vi "数据处理整合 (子VI).vi"(11 "枚举":enum16{"实时数据排序", "小时数据排序"}(ring)) -> (3 "已排序的数组":string[](array[string]))   [LabVIEW 2016, in "数据传输系统.lvlib"]
uses:
  <userlib>/_OpenG.lib/array/array.llb/Remove Duplicates from 1D Array (String)__ogtk.vi
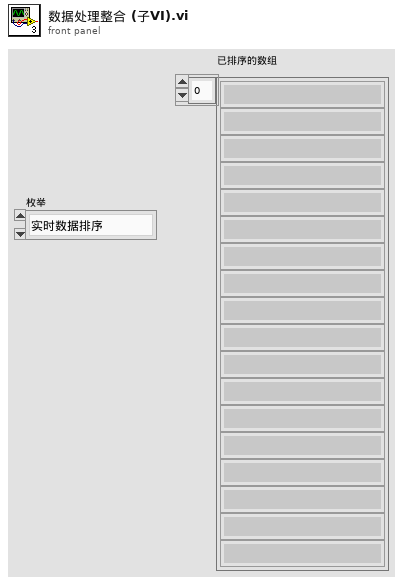
[diagram p1: front panel]
types:
  T1 = cluster{"PH":string[][], "CODCr":string[][], "氨氮":string[][], "CODMn":string[][], "总氮":string[][], "总磷":string[][], "电导率":string[][], "水温":string[][], "DO":string[][], "浊度":string[][], "叶绿素":string[][], "藻密度":string[][], "铜":string[][], "盐度":string[][], "水位":string[][], "流速":string[][], "瞬时流量":string[][], "累积流量":string[][], "亚硝酸盐":string[][], "硫化物":string[][], "ORP":string[][], "铅":string[][], "镉":string[][], "锌":string[][], "镍":string[][], "锰":string[][], "汞":string[][]}
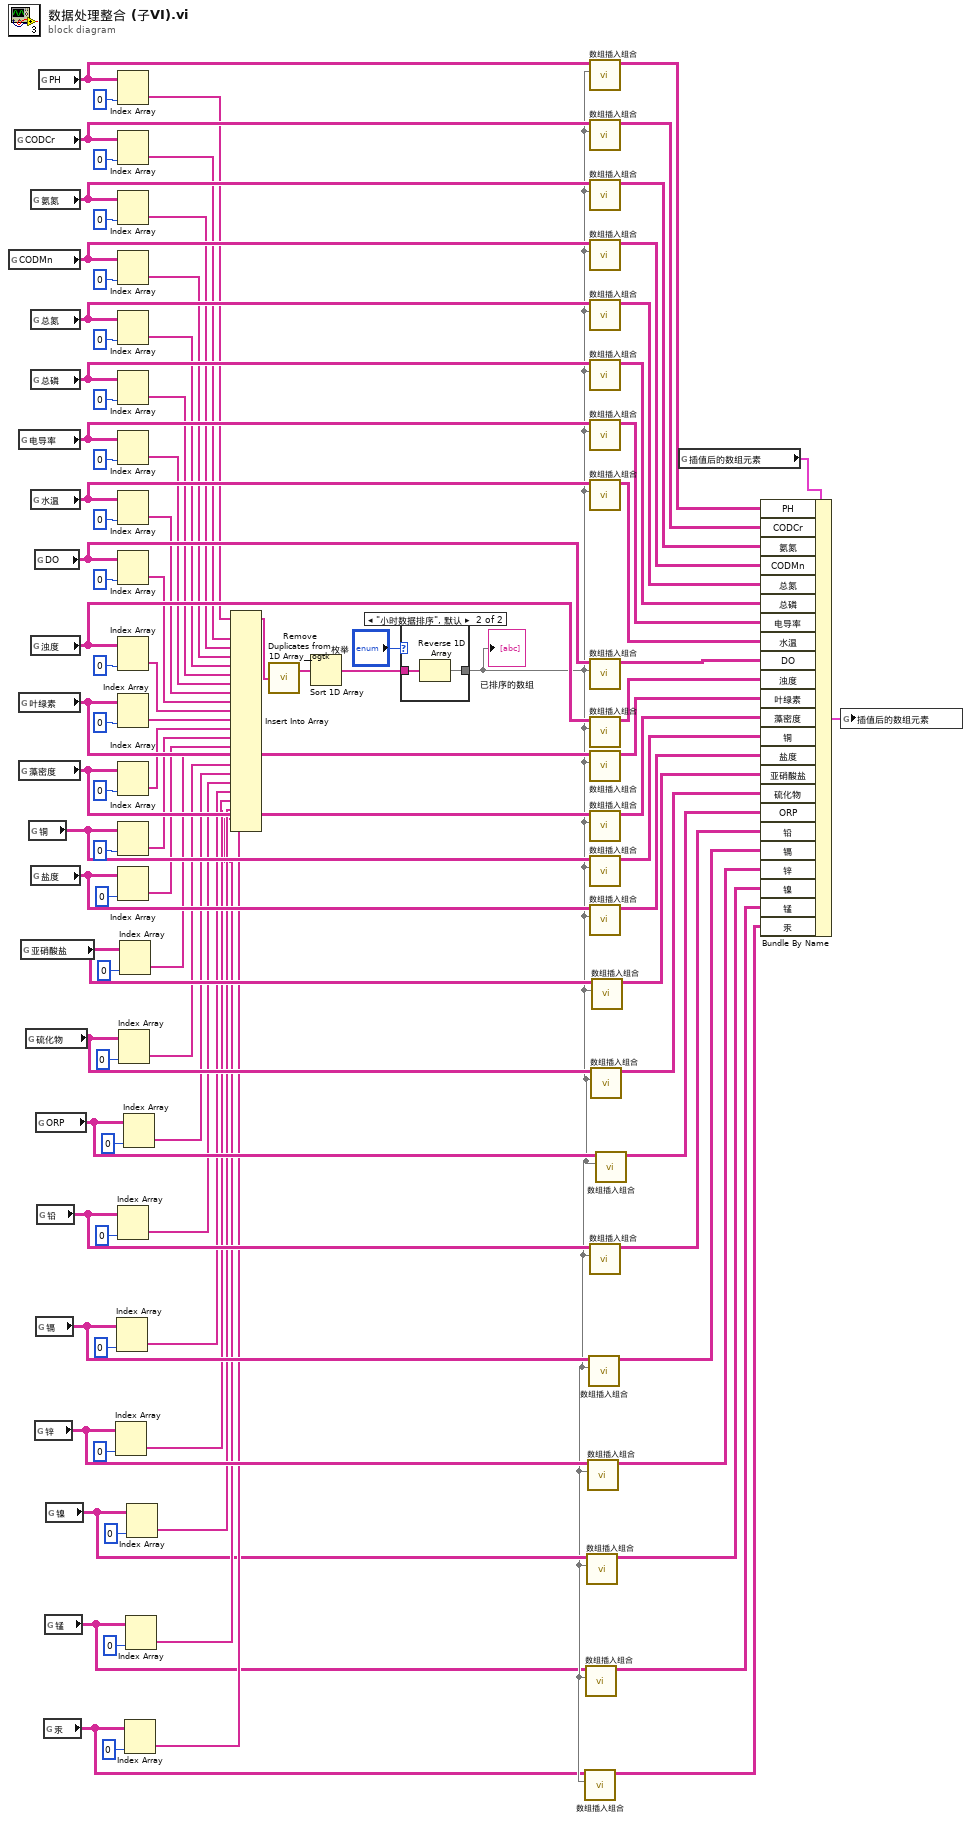
[diagram p0: block diagram]
diagram:
  n1 = global read "全局 所有参数.vi" "CODMn"() -> (w80:string[][])
  n2 = global read "全局 所有参数.vi" "CODCr"() -> (w78:string[][])
  n3 = global read "全局 所有参数.vi" "电导率"() -> (w83:string[][])
  n4 = global read "全局 所有参数.vi" "叶绿素"() -> (w87:string[][])
  n5 = global read "全局 所有参数.vi" "藻密度"() -> (w88:string[][])
  n6 = global read "全局 所有参数.vi" "亚硝酸盐"() -> (w37:string[][])
  n7 = global read "全局 所有参数.vi" "硫化物"() -> (w36:string[][])
  n8 = global read "全局 所有参数.vi" "铜"() -> (w47:string[][])
  n9 = global read "全局 所有参数.vi" "氨氮"() -> (w79:string[][])
  n10 = global read "全局 所有参数.vi" "总氮"() -> (w81:string[][])
  n11 = global read "全局 所有参数.vi" "总磷"() -> (w82:string[][])
  n12 = global read "全局 所有参数.vi" "水温"() -> (w84:string[][])
  n13 = global read "全局 所有参数.vi" "浊度"() -> (w86:string[][])
  n14 = global read "全局 所有参数.vi" "盐度"() -> (w46:string[][])
  n15 = global read "全局 所有参数.vi" "DO"() -> (w85:string[][])
  n16 = global read "全局 所有参数.vi" "锌"() -> (w21:string[][])
  n17 = global read "全局 所有参数.vi" "ORP"() -> (w33:string[][])
  n18 = global read "全局 所有参数.vi" "镉"() -> (w22:string[][])
  n19 = global read "全局 所有参数.vi" "铅"() -> (w25:string[][])
  n20 = global read "全局 所有参数.vi" "PH"() -> (w76:string[][])
  n21 = global read "全局 所有参数.vi" "汞"() -> (w4:string[][])
  n22 = global read "全局 所有参数.vi" "锰"() -> (w5:string[][])
  n23 = global read "全局 所有参数.vi" "镍"() -> (w7:string[][])
  n24 = Index Array(array=w21, index (col)=0 ("索引 (行)")) -> (element=w14:string[])  [unwired: 1 in]
  n25 = Index Array(array=w22, index (col)=0 ("索引 (行)")) -> (element=w15:string[])  [unwired: 1 in]
  n26 = Index Array(array=w76, index (col)=0 ("索引 (行)")) -> (element=w63:string[])  [unwired: 1 in]
  n27 = Index Array(array=w78, index (col)=0 ("索引 (行)")) -> (element=w64:string[])  [unwired: 1 in]
  n28 = Index Array(array=w79, index (col)=0 ("索引 (行)")) -> (element=w65:string[])  [unwired: 1 in]
  n29 = Index Array(array=w80, index (col)=0 ("索引 (行)")) -> (element=w66:string[])  [unwired: 1 in]
  n30 = Index Array(array=w81, index (col)=0 ("索引 (行)")) -> (element=w67:string[])  [unwired: 1 in]
  n31 = Index Array(array=w82, index (col)=0 ("索引 (行)")) -> (element=w68:string[])  [unwired: 1 in]
  n32 = Index Array(array=w83, index (col)=0 ("索引 (行)")) -> (element=w69:string[])  [unwired: 1 in]
  n33 = Index Array(array=w84, index (col)=0 ("索引 (行)")) -> (element=w70:string[])  [unwired: 1 in]
  n34 = Index Array(array=w85, index (col)=0 ("索引 (行)")) -> (element=w71:string[])  [unwired: 1 in]
  n35 = Index Array(array=w86, index (col)=0 ("索引 (行)")) -> (element=w72:string[])  [unwired: 1 in]
  n36 = Index Array(array=w87, index (col)=0 ("索引 (行)")) -> (element=w73:string[])  [unwired: 1 in]
  n37 = Index Array(array=w88, index (col)=0 ("索引 (行)")) -> (element=w74:string[])  [unwired: 1 in]
  n38 = Index Array(array=w47, index (col)=0 ("索引 (行)")) -> (element=w45:string[])  [unwired: 1 in]
  n39 = Index Array(array=w46, index (col)=0 ("索引 (行)")) -> (element=w44:string[])  [unwired: 1 in]
  n40 = Index Array(array=w25, index (col)=0 ("索引 (行)")) -> (element=w16:string[])  [unwired: 1 in]
  n41 = Index Array(array=w36, index (col)=0 ("索引 (行)")) -> (element=w28:string[])  [unwired: 1 in]
  n42 = Index Array(array=w37, index (col)=0 ("索引 (行)")) -> (element=w27:string[])  [unwired: 1 in]
  n43 = Index Array(array=w33, index (col)=0 ("索引 (行)")) -> (element=w29:string[])  [unwired: 1 in]
  n44 = Index Array(array=w4, index (col)=0 ("索引 (行)")) -> (element=w8:string[])  [unwired: 1 in]
  n45 = Index Array(array=w5, index (col)=0 ("索引 (行)")) -> (element=w9:string[])  [unwired: 1 in]
  n46 = Index Array(array=w7, index (col)=0 ("索引 (行)")) -> (element=w10:string[])  [unwired: 1 in]
  n47 = Insert Into Array(array=w63, new element #1=w64, new element #2=w65, new element #3=w66, new element #4=w67, new element #5=w68, new element #6=w69, new element #7=w70, new element #8=w71, new element #9=w72, new element #10=w73, new element #11=w74, new element #12=w45, new element #13=w44, new element #14=w27, new element #15=w28, new element #16=w29, new element #17=w16, new element #18=w15, new element #19=w14, new element #20=w10, new element #21=w9, new element #22=w8) -> (w75:string[])  [unwired: 1 in]
  n48 = call-poly <userlib>:"Remove Duplicates from 1D Array__ogtk.vi"("Input Array"=w75) -> ("Output Array"=w62:string[])  [unwired: 1 out]
  n49 = Sort 1D Array(array=w62) -> (sorted array=w48:string[])
  n50 = case shown="\"小时数据排序\", 默认" "枚举" {
    tunnel: w48 -> [w100 w102]
    tunnel: [w100 w101] -> w6
    frame "实时数据排序" {
    }
    frame "小时数据排序", Default {
      n51 = Reverse 1D Array(array=w102) -> (reversed array=w101:string[])
    }
  }
  "已排序的数组" <- w6
  n52 = call "数组插入组合.vi"("排序后的一维数组"=w6, "输入数组"=w4) -> ("输出结果"=w1:string[][])  [unwired: 9 in]
  n53 = call "数组插入组合.vi"("排序后的一维数组"=w6, "输入数组"=w5) -> ("输出结果"=w2:string[][])  [unwired: 9 in]
  n54 = call "数组插入组合.vi"("排序后的一维数组"=w6, "输入数组"=w7) -> ("输出结果"=w3:string[][])  [unwired: 9 in]
  n55 = call "数组插入组合.vi"("排序后的一维数组"=w6, "输入数组"=w21) -> ("输出结果"=w17:string[][])  [unwired: 9 in]
  n56 = call "数组插入组合.vi"("排序后的一维数组"=w6, "输入数组"=w22) -> ("输出结果"=w18:string[][])  [unwired: 9 in]
  n57 = call "数组插入组合.vi"("排序后的一维数组"=w6, "输入数组"=w76) -> ("输出结果"=w77:string[][])  [unwired: 9 in]
  n58 = call "数组插入组合.vi"("排序后的一维数组"=w6, "输入数组"=w78) -> ("输出结果"=w89:string[][])  [unwired: 9 in]
  n59 = call "数组插入组合.vi"("排序后的一维数组"=w6, "输入数组"=w79) -> ("输出结果"=w90:string[][])  [unwired: 9 in]
  n60 = call "数组插入组合.vi"("排序后的一维数组"=w6, "输入数组"=w80) -> ("输出结果"=w91:string[][])  [unwired: 9 in]
  n61 = call "数组插入组合.vi"("排序后的一维数组"=w6, "输入数组"=w81) -> ("输出结果"=w92:string[][])  [unwired: 9 in]
  n62 = call "数组插入组合.vi"("排序后的一维数组"=w6, "输入数组"=w82) -> ("输出结果"=w93:string[][])  [unwired: 9 in]
  n63 = call "数组插入组合.vi"("排序后的一维数组"=w6, "输入数组"=w83) -> ("输出结果"=w94:string[][])  [unwired: 9 in]
  n64 = call "数组插入组合.vi"("排序后的一维数组"=w6, "输入数组"=w84) -> ("输出结果"=w95:string[][])  [unwired: 9 in]
  n65 = call "数组插入组合.vi"("排序后的一维数组"=w6, "输入数组"=w85) -> ("输出结果"=w96:string[][])  [unwired: 9 in]
  n66 = call "数组插入组合.vi"("排序后的一维数组"=w6, "输入数组"=w86) -> ("输出结果"=w97:string[][])  [unwired: 9 in]
  n67 = call "数组插入组合.vi"("排序后的一维数组"=w6, "输入数组"=w87) -> ("输出结果"=w98:string[][])  [unwired: 9 in]
  n68 = call "数组插入组合.vi"("排序后的一维数组"=w6, "输入数组"=w88) -> ("输出结果"=w99:string[][])  [unwired: 9 in]
  n69 = call "数组插入组合.vi"("排序后的一维数组"=w6, "输入数组"=w47) -> ("输出结果"=w43:string[][])  [unwired: 9 in]
  n70 = call "数组插入组合.vi"("排序后的一维数组"=w6, "输入数组"=w46) -> ("输出结果"=w42:string[][])  [unwired: 9 in]
  n71 = call "数组插入组合.vi"("排序后的一维数组"=w6, "输入数组"=w25) -> ("输出结果"=w19:string[][])  [unwired: 9 in]
  n72 = call "数组插入组合.vi"("排序后的一维数组"=w6, "输入数组"=w36) -> ("输出结果"=w30:string[][])  [unwired: 9 in]
  n73 = call "数组插入组合.vi"("排序后的一维数组"=w6, "输入数组"=w37) -> ("输出结果"=w32:string[][])  [unwired: 9 in]
  n74 = call "数组插入组合.vi"("排序后的一维数组"=w6, "输入数组"=w33) -> ("输出结果"=w31:string[][])  [unwired: 9 in]
  n75 = global read "插值后的新数组.vi" "插值后的数组元素"() -> (w39:T1)
  n76 = Bundle By Name(cluster=w39, "PH"=w77, "CODCr"=w89, "氨氮"=w90, "CODMn"=w91, "总氮"=w92, "总磷"=w93, "电导率"=w94, "水温"=w95, "DO"=w96, "浊度"=w97, "叶绿素"=w98, "藻密度"=w99, "铜"=w43, "盐度"=w42, "亚硝酸盐"=w32, "硫化物"=w30, "ORP"=w31, "铅"=w19, "镉"=w18, "锌"=w17, "镍"=w3, "锰"=w2, "汞"=w1) -> (w26:T1)
  n77 = global write "插值后的新数组.vi" "插值后的数组元素"(w26) -> ()
